vi "8257D_VI.vi"(3 "PowerLevel":dbl, 4 "Frequency":dbl, 5 "8257D":refnum<visa-resource-name>) -> ()   [LabVIEW 2017]
panel:
  in  "AgilentRfSigGenLib.IAgilentRfSigGen4":refnum<k7>
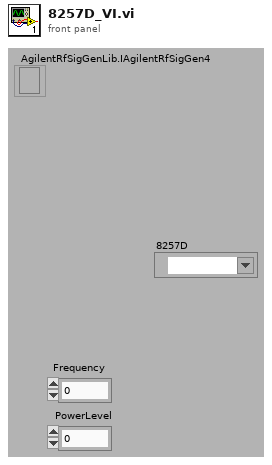
[diagram p1: front panel]
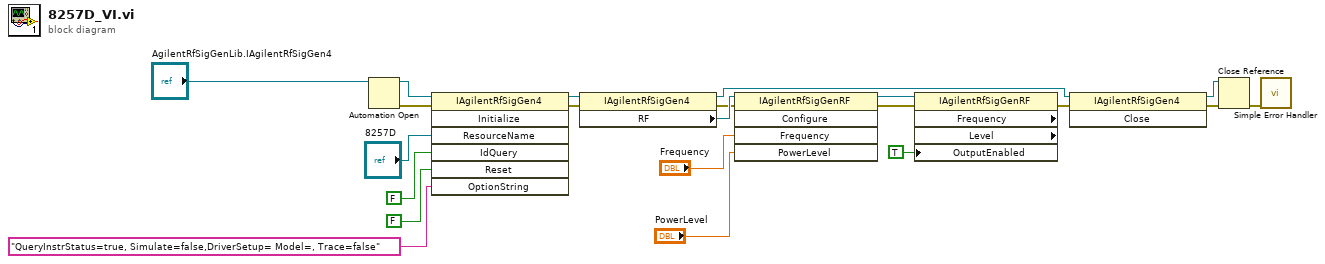
[diagram p0: block diagram]
diagram:
  n1 = Automation Open(Automation Refnum="AgilentRfSigGenLib.IAgilentRfSigGen4") -> (Automation Refnum=w11:refnum<k7>, error out=w19:errorcluster)  [unwired: 3 in]
  n2 = invoke class="IAgilentRfSigGen4" method="Initialize"(reference=w11, error in=w19, "ResourceName"="8257D", "IdQuery"=FALSE, "Reset"=FALSE, "OptionString"="QueryInstrStatus=true, Simulate=false,DriverSetup= Model=, Trace=false") -> (reference out=w8:refnum<k7>, error out=w7:errorcluster)  [unwired: 1 in, 5 out]
  n3 = property class="IAgilentRfSigGen4"(reference=w8, error in=w7) -> (reference out=w5:refnum<k7>, error out=w17:errorcluster, "RF"=w18:refnum<k7>)
  n4 = invoke class="IAgilentRfSigGenRF" method="Configure"(reference=w18, error in=w17, "Frequency"="Frequency", "PowerLevel"="PowerLevel") -> (reference out=w4:refnum<k7>, error out=w3:errorcluster)  [unwired: 1 in, 3 out]
  n5 = property class="IAgilentRfSigGenRF" props=["Frequency", "Level", "OutputEnabled"](reference=w4, error in=w3, "OutputEnabled"=TRUE) -> (error out=w2:errorcluster)  [unwired: 3 out]
  n6 = invoke class="IAgilentRfSigGen4" method="Close"(reference=w5, error in=w2) -> (reference out=w14:refnum<k7>, error out=w13:errorcluster)  [unwired: 1 in, 1 out]
  n7 = Close Reference(reference=w14, error in (no error)=w13) -> (error out=w10:errorcluster)
  n8 = call <vilib>:"Simple Error Handler.vi"("error in (no error)"=w10) -> ()  [unwired: 4 in, 5 out]
